vi "Test Assert Array Equivalent.vi"(8 "error in (no error)":errorcluster) -> (0 "error out":errorcluster)   [LabVIEW 2013]
uses:
  classes/Assert/Assert.lvclass
  classes/Test/Test.lvclass
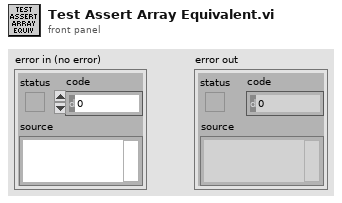
[diagram p1: front panel]
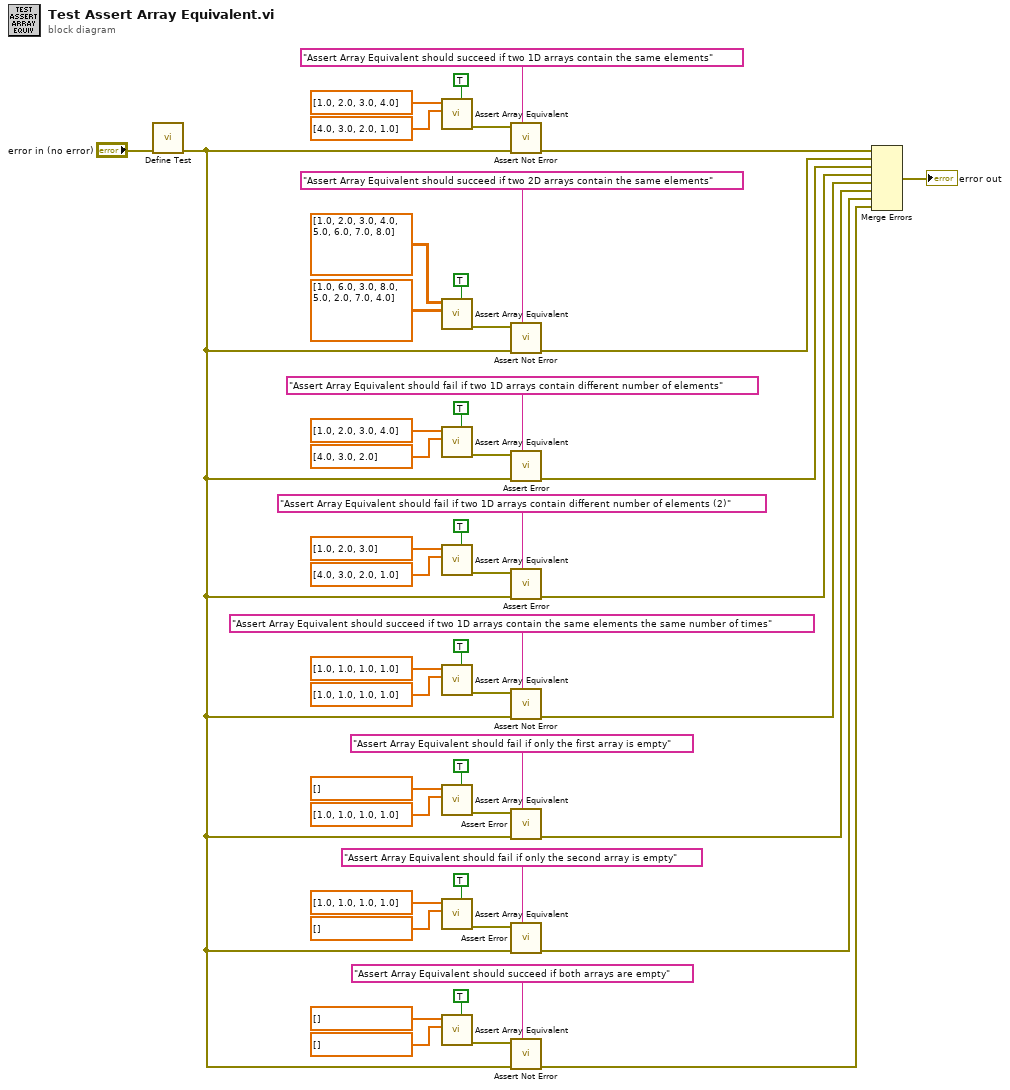
[diagram p0: block diagram]
diagram:
  n1 = call "Define Test.vi"("error in (no error)"="error in (no error)") -> ("error out"=w2:errorcluster)  [unwired: 9 in, 1 out]
  n2 = call "Assert Array Equivalent.vi"("Assert Only? (F)"=TRUE, "Second Array"=dbl[] [4.0, 3.0, 2.0, 1.0] ("initialized array"), "First Array"=dbl[] [1.0, 2.0, 3.0, 4.0] ("initialized array")) -> ("error out"=w51:errorcluster)  [unwired: 7 in, 1 out]
  n3 = call "Assert Array Equivalent.vi"("Assert Only? (F)"=TRUE, "Second Array"=dbl[][] [[1.0, 6.0, 3.0, 8.0], [5.0, 2.0, 7.0, 4.0]] ("initialized array"), "First Array"=dbl[][] [[1.0, 2.0, 3.0, 4.0], [5.0, 6.0, 7.0, 8.0]] ("initialized array")) -> ("error out"=w39:errorcluster)  [unwired: 7 in, 1 out]
  n4 = call "Assert Array Equivalent.vi"("Assert Only? (F)"=TRUE, "Second Array"=dbl[] [4.0, 3.0, 2.0] ("initialized array"), "First Array"=dbl[] [1.0, 2.0, 3.0, 4.0] ("initialized array")) -> ("error out"=w33:errorcluster)  [unwired: 7 in, 1 out]
  n5 = call "Assert Array Equivalent.vi"("Assert Only? (F)"=TRUE, "Second Array"=dbl[] [4.0, 3.0, 2.0, 1.0] ("initialized array"), "First Array"=dbl[] [1.0, 2.0, 3.0] ("initialized array")) -> ("error out"=w31:errorcluster)  [unwired: 7 in, 1 out]
  n6 = call "Assert Array Equivalent.vi"("Assert Only? (F)"=TRUE, "Second Array"=dbl[] [1.0, 1.0, 1.0, 1.0] ("initialized array"), "First Array"=dbl[] [1.0, 1.0, 1.0, 1.0] ("initialized array")) -> ("error out"=w21:errorcluster)  [unwired: 7 in, 1 out]
  n7 = call "Assert Array Equivalent.vi"("Assert Only? (F)"=TRUE, "Second Array"=dbl[] [1.0, 1.0, 1.0, 1.0] ("initialized array"), "First Array"=dbl[] [] ("initialized array")) -> ("error out"=w19:errorcluster)  [unwired: 7 in, 1 out]
  n8 = call "Assert Array Equivalent.vi"("Assert Only? (F)"=TRUE, "Second Array"=dbl[] [] ("initialized array"), "First Array"=dbl[] [1.0, 1.0, 1.0, 1.0] ("initialized array")) -> ("error out"=w13:errorcluster)  [unwired: 7 in, 1 out]
  n9 = call "Assert Array Equivalent.vi"("Assert Only? (F)"=TRUE, "Second Array"=dbl[] [] ("initialized array"), "First Array"=dbl[] [] ("initialized array")) -> ("error out"=w3:errorcluster)  [unwired: 7 in, 1 out]
  n10 = call "Assert Not Error.vi"("Label"="Assert Array Equivalent should succeed if two 1D arrays contain the same elements", "error in (no error)"=w2, "Not Error?"=w51) -> ("error out"=w47:errorcluster)  [unwired: 7 in, 1 out]
  n11 = call "Assert Not Error.vi"("Label"="Assert Array Equivalent should succeed if two 2D arrays contain the same elements", "error in (no error)"=w2, "Not Error?"=w39) -> ("error out"=w38:errorcluster)  [unwired: 7 in, 1 out]
  n12 = call "Assert Error.vi"("Label"="Assert Array Equivalent should fail if two 1D arrays contain different number of elements", "error in (no error)"=w2, "Error?"=w33) -> ("error out"=w32:errorcluster)  [unwired: 7 in, 1 out]
  n13 = call "Assert Error.vi"("Label"="Assert Array Equivalent should fail if two 1D arrays contain different number of elements (2)", "error in (no error)"=w2, "Error?"=w31) -> ("error out"=w26:errorcluster)  [unwired: 7 in, 1 out]
  n14 = call "Assert Not Error.vi"("Label"="Assert Array Equivalent should succeed if two 1D arrays contain the same elements the same number of times", "error in (no error)"=w2, "Not Error?"=w21) -> ("error out"=w20:errorcluster)  [unwired: 7 in, 1 out]
  n15 = call "Assert Error.vi"("Label"="Assert Array Equivalent should fail if only the first array is empty", "error in (no error)"=w2, "Error?"=w19) -> ("error out"=w14:errorcluster)  [unwired: 7 in, 1 out]
  n16 = call "Assert Error.vi"("Label"="Assert Array Equivalent should fail if only the second array is empty", "error in (no error)"=w2, "Error?"=w13) -> ("error out"=w8:errorcluster)  [unwired: 7 in, 1 out]
  n17 = call "Assert Not Error.vi"("Label"="Assert Array Equivalent should succeed if both arrays are empty", "error in (no error)"=w2, "Not Error?"=w3) -> ("error out"=w1:errorcluster)  [unwired: 7 in, 1 out]
  n18 = Merge Errors(w47, w38, w32, w26, w20, w14, w8, w1) -> (→"error out":errorcluster)
